vi "Driving with the Limelight search and aim.vi"(8 "error in (no error)":errorcluster) -> (0 "TurnCommand":dbl(knob)=nan scale=-1.0..1.0, 1 "SpeedCommand":dbl(knob)=-0.0 scale=0.0..1.0, 3 "TargetValid":bool)   [LabVIEW 2019]
uses:
  Framework/Robot Global Data.vi
  <vilib>/addons/control/pid/NI_PID_pid.lvlib
  <vilib>/addons/control/pid/pid.llb/PID (DBL).vi
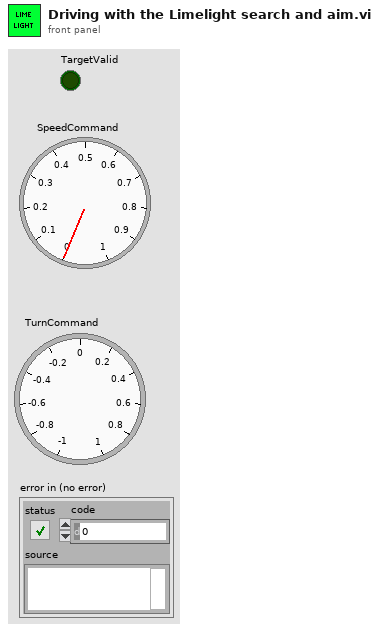
[diagram p1: front panel]
types:
  T1 = cluster{"proportional gain (Kc)":dbl, "integral time (Ti, min)":dbl, "derivative time (Td, min)":dbl}
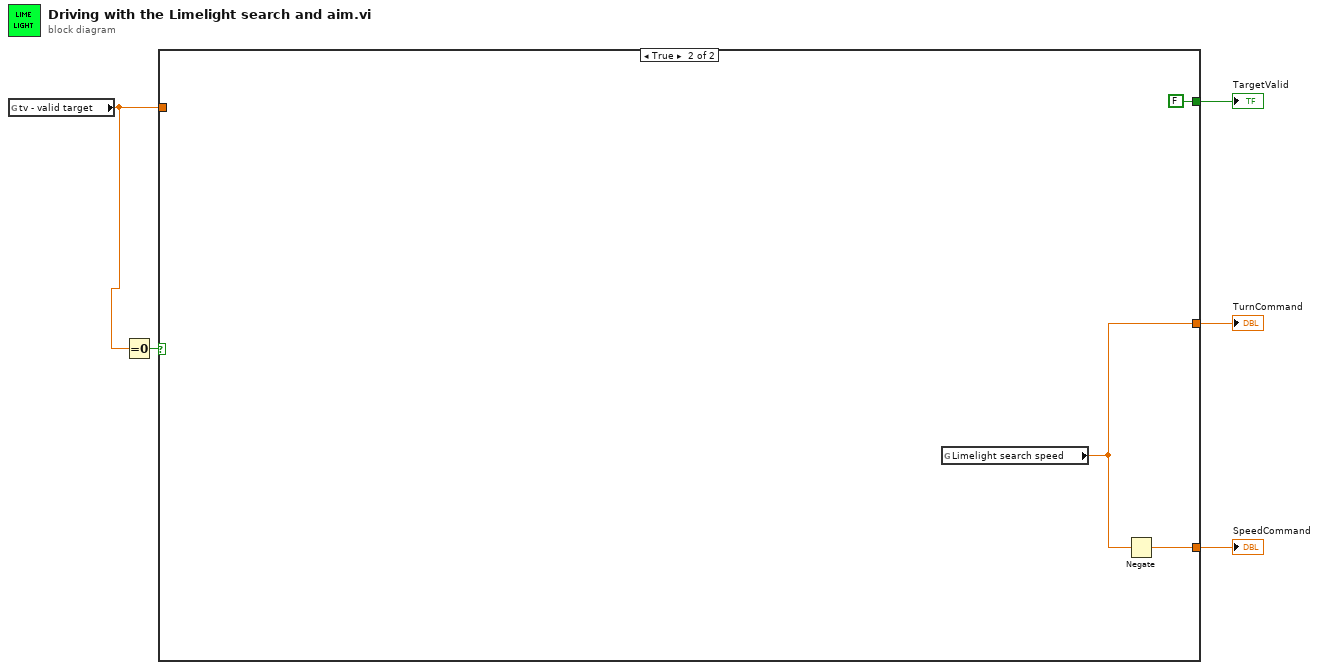
[diagram p0: block diagram]
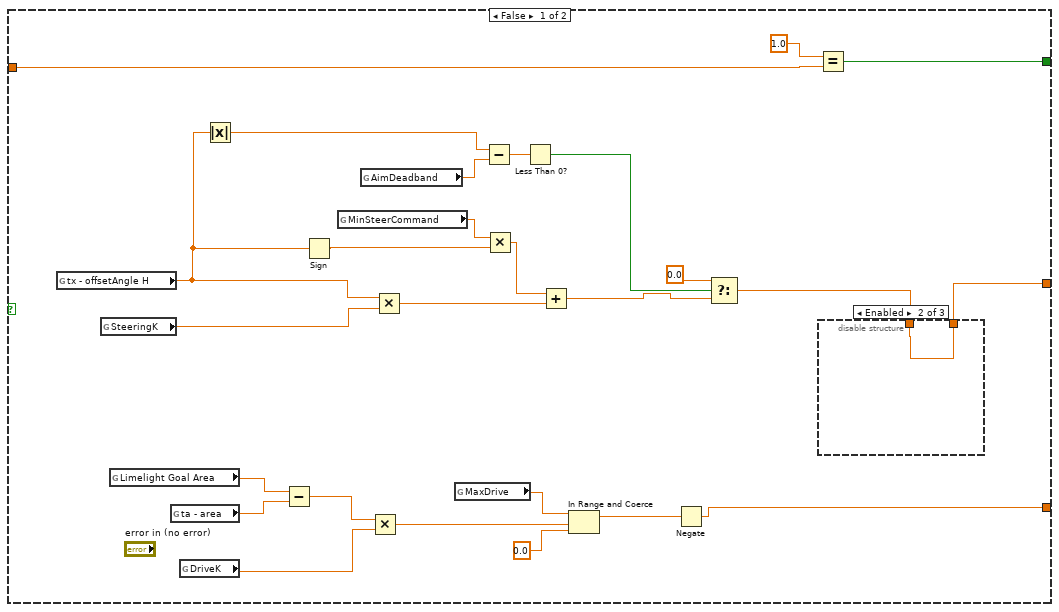
[diagram p2: hidden frame]
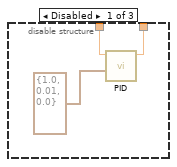
[diagram p3: hidden frame]
diagram:
  n1 = global read "Robot Global Data.vi" "tv - valid target"() -> (w1:dbl)
  n2 = Equal To 0?(x=w1) -> (x = 0?=w2:bool)
  n3 = case shown="True" w2 {
    tunnel: [w19 w36] -> w5
    tunnel: [w17 FALSE] -> w4
    tunnel: w1 -> [w14 _]
    tunnel: [w7 w37] -> w3
    frame False {
      n4 = global read "Robot Global Data.vi" "tx - offsetAngle H"() -> (w16:dbl)
      n5 = global read "Robot Global Data.vi" "SteeringK"() -> (w10:dbl)
      n6 = global read "Robot Global Data.vi" "Limelight Goal Area"() -> (w11:dbl)
      n7 = global read "Robot Global Data.vi" "ta - area"() -> (w15:dbl)
      n8 = global read "Robot Global Data.vi" "DriveK"() -> (w12:dbl)
      n9 = Absolute Value(x=w16) -> (abs(x)=w28:dbl)
      n10 = Subtract(x=w11, y=w15) -> (x-y=w23:dbl)
      n11 = Sign(1:w16) -> (0:w24:dbl)
      n12 = global read "Robot Global Data.vi" "MinSteerCommand"() -> (w8:dbl)
      n13 = global read "Robot Global Data.vi" "AimDeadband"() -> (w9:dbl)
      n14 = Multiply(x=w23, y=w12) -> (x*y=w22:dbl)
      n15 = Multiply(x=w16, y=w10) -> (x*y=w26:dbl)
      n16 = global read "Robot Global Data.vi" "MaxDrive"() -> (w13:dbl)
      n17 = Subtract(x=w28, y=w9) -> (x-y=w29:dbl)
      n18 = Multiply(x=w8, y=w24) -> (x*y=w27:dbl)
      n19 = Less Than 0?(x=w29) -> (x < 0?=w30:bool)
      n20 = Add(x=w27, y=w26) -> (x+y=w6:dbl)
      n21 = In Range and Coerce(upper limit=w13, x=w22, lower limit=0.0) -> (coerced(x)=w20:dbl)  [unwired: 1 out]
      n22 = Negate(x=w20) -> (-x=w19:dbl)
      n23 = Select(t=0.0, s=w30, f=w6) -> (s? t:f=w25:dbl)
      n24 = Equal?(x=1.0, y=w14) -> (x = y?=w17:bool)
      n25 = disable-structure shown="Enabled" {
        disable-tunnel: w25 -> [w34 w35 _]
        disable-tunnel: [w33 w35 _] -> w7
        frame Disabled {
          n26 = call-poly <vilib>:"PID.vi"("PID gains"=T1 {"proportional gain (Kc)"=1.0, "integral time (Ti, min)"=0.01, "derivative time (Td, min)"=0.0}, "setpoint"=w34) -> ("output"=w33:dbl)  [unwired: 8 in, 1 out]
        }
        frame Enabled {
        }
        frame Disabled {
        }
      }
    }
    frame True {
      n27 = global read "Robot Global Data.vi" "Limelight search speed"() -> (w37:dbl)
      n28 = Negate(x=w37) -> (-x=w36:dbl)
    }
  }
  "TurnCommand" <- w3
  "SpeedCommand" <- w5
  "TargetValid" <- w4
